vi "Data Thread.vi"() -> ()   [LabVIEW 2016]
doc: "数据处理线程；\n硬件采集的原始数据经DAQData数据队列传输至此线程，计算后获得所有物理通道数据、虚拟通道数据，再分发给显示线程数据队列（DispDATA）以及存储线程数据队列（SaveDATA）"
uses:
  ToolKit/Formula/Ctrls/PSFormula_FOR_Formula Node.ctl
  ToolKit/Formula/Ctrls/PSFormula_FOR_Formula Step.ctl
  ToolKit/Formula/Ctrls/PSFormula_FOR_Formula Para.ctl
  ToolKit/Formula/Ctrls/PSFormula_FOR_Formula MidVar Data.ctl
  HardWare/Ctrls/HardWare _ Data Queue Manage FGV Operation.ctl
  X-DAQ Viewer/Controls/ConfigFGVCtrl.ctl
  <vilib>/Analysis/baseanly.llb/Mean (DBL).vi
  Architecture/Queue Management/ARC_Queue Create_Single.vi
  Architecture/Queue Management/ARC_Queue Remove Element.vi
  Architecture/Queue Management/ARC_Queue Valid.vi
  Ctrls/GlobeVaribles.vi
  Architecture/Queue Management/ARC_Queue Insert Element.vi
  <vilib>/Utility/error.llb/DialogType.ctl
  <vilib>/Analysis/NI_AALBase.lvlib
panel:
  in  "Parameter":cluster{"Q-Local":string, "Variant":variant}
  in  "TempVariable":T5
  out "Error Report":string
  out "Current State":string
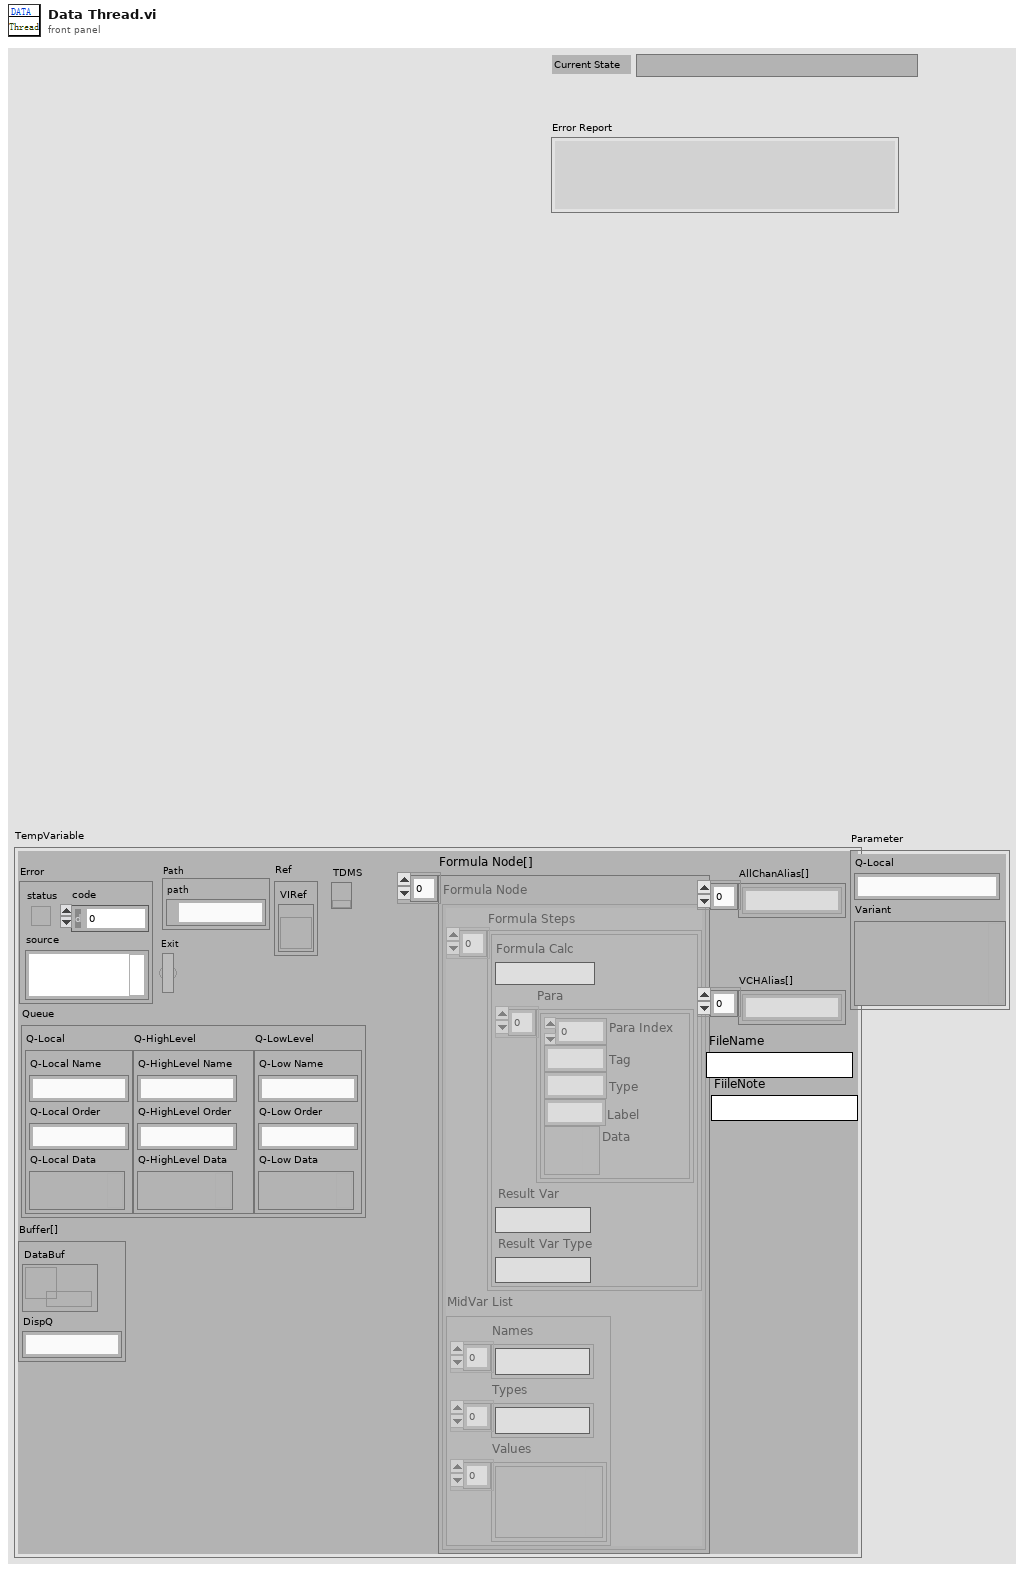
[diagram p1: front panel]
types:
  T1 = typedef "PSFormula_FOR_Formula Node.ctl" = cluster{"Formula Steps":T2[], "MidVar List":T4}
  T2 = typedef "PSFormula_FOR_Formula Step.ctl" = cluster{"Formula Calc":string, "Para":T3[], "Result Var":string, "Result Var Type":string}
  T3 = typedef "PSFormula_FOR_Formula Para.ctl" = cluster{"Para Index":i32, "Tag":string, "Type":string, "Label":string, "Data":variant}
  T4 = typedef "PSFormula_FOR_Formula MidVar Data.ctl" = cluster{"Names":string[], "Types":string[], "Values":variant[]}
  T5 = cluster{"Error":errorcluster, "Exit":bool, "Path":cluster{"path":path}, "Ref":cluster{"VIRef":refnum<vi>}, "Queue":cluster{"Q-Local":cluster{"Q-Local Name":string, "Q-Local Order":string, "Q-Local Data":variant}, "Q-HighLevel":cluster{"Q-HighLevel Name":string, "Q-HighLevel Order":string, "Q-HighLevel Data":variant}, "Q-LowLevel":cluster{"Q-Low Name":string, "Q-Low Order":string, "Q-Low Data":variant}}, "Formula Node[]":T1[], "Buffer[]":cluster{"DataBuf":refnum<queue>, "DispQ":string}, "TDMS":refnum<k34>, "AllChanAlias[]":string[], "VCHAlias[]":string[], "FileName":string, "FiileNote":string}
  T6 = cluster{"LocalName":string, "DataBuf":refnum<queue>}
  T7 = typedef "ConfigFGVCtrl.ctl" = enum16{"Initialize", "Get Value", "Set Value", "Search Info"}
  T8 = typedef "HardWare _ Data Queue Manage FGV Operation.ctl" = enum16{"Initialize", "Add", "Read", "All"}
  T9 = enum16{"Obtain Notifier", "Send Notification", "Wait Notification", "Release Notifier"}
  T10 = typedef "DialogType.ctl" = u16
  T11 = typedef "HardWare _ Channel Info.ctl" = cluster{"PhyCHtags[]":string[], "VCHTags":string[], "AllNames":string[], "AllAlias":string[], "AllUnits":string[], "AllName(Unit)":string[], "AllAlarmMax":dbl[], "AllAlarmMin":dbl[], "VCHFormula[]":string[], "VCHAlias[]":string[]}
  T12 = cluster{"PhyCHtags[]":string[], "AllAlias":string[]}
  T13 = typedef "Continuous Operations.ctl" = enum16{"Writting", "Pause", "Stop"}
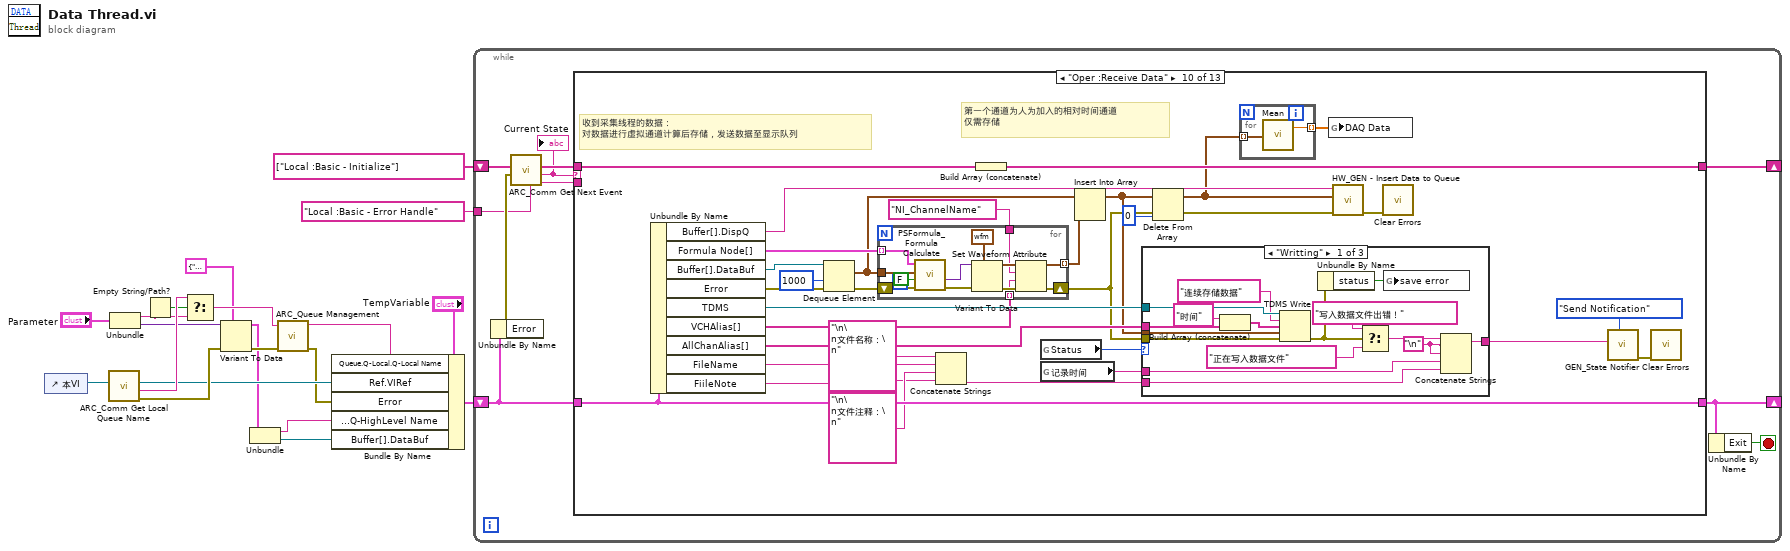
[diagram p0: block diagram]
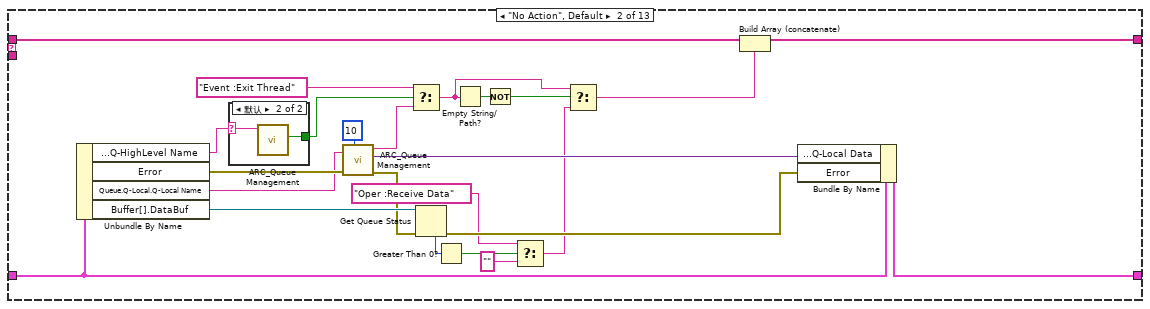
[diagram p3: hidden frame]
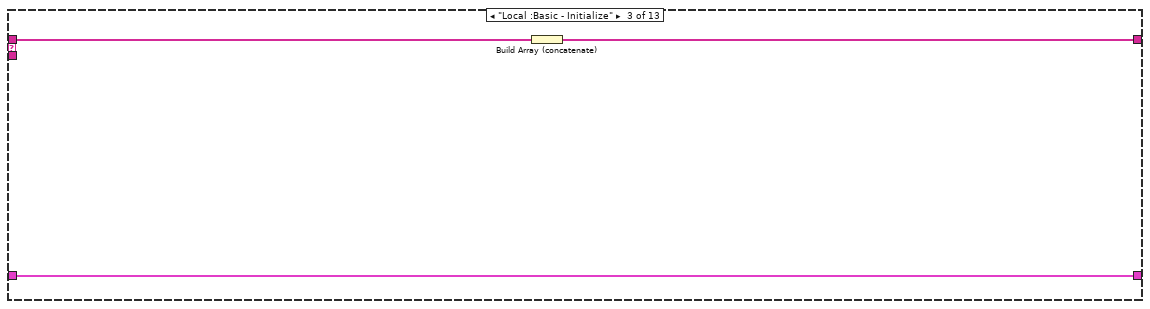
[diagram p5: hidden frame]
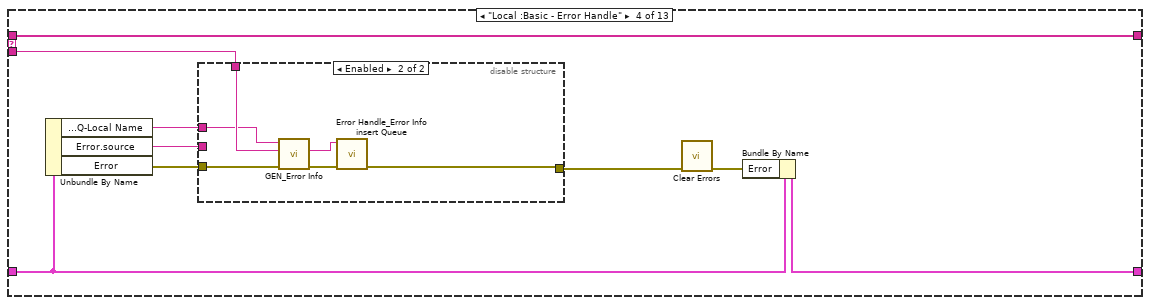
[diagram p6: hidden frame]
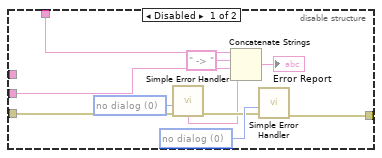
[diagram p7: hidden frame]
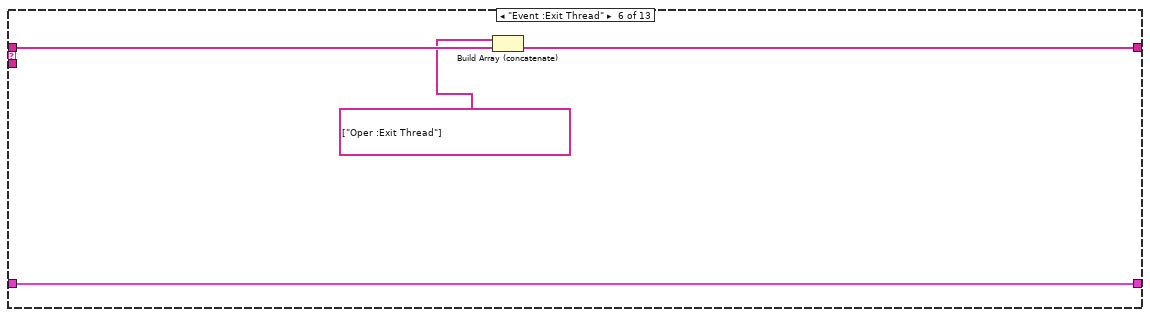
[diagram p9: hidden frame]
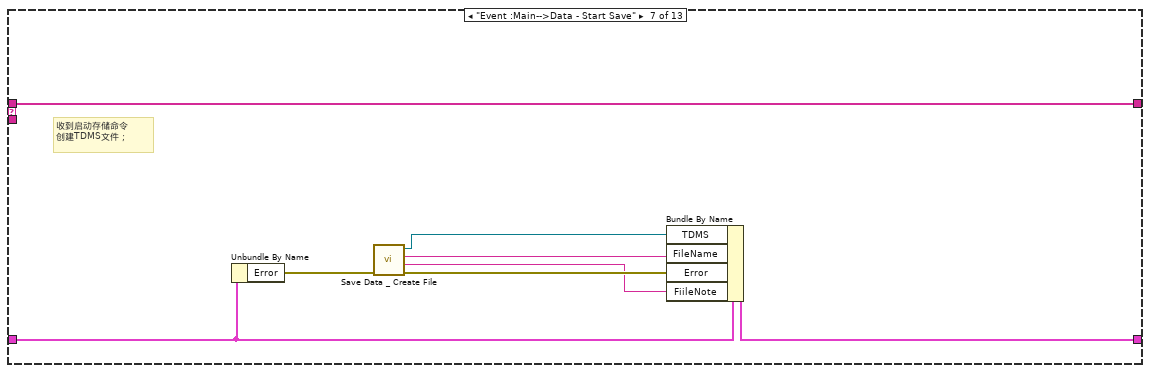
[diagram p10: hidden frame]
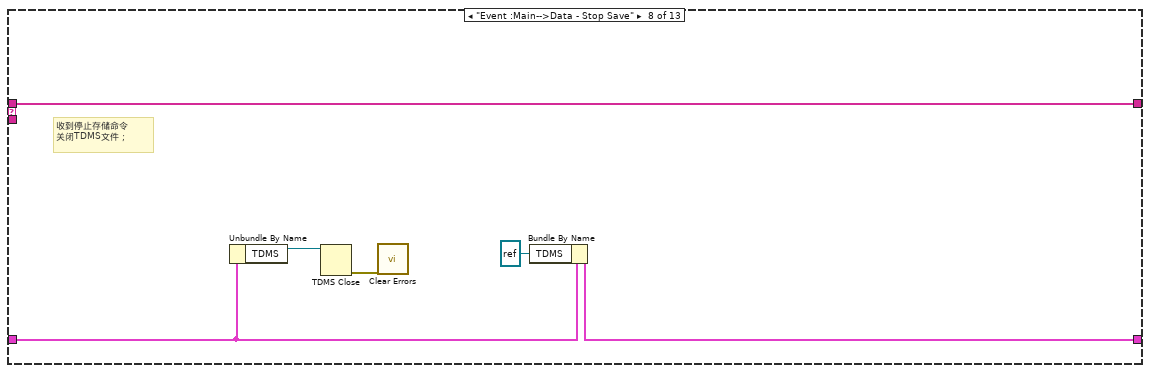
[diagram p11: hidden frame]
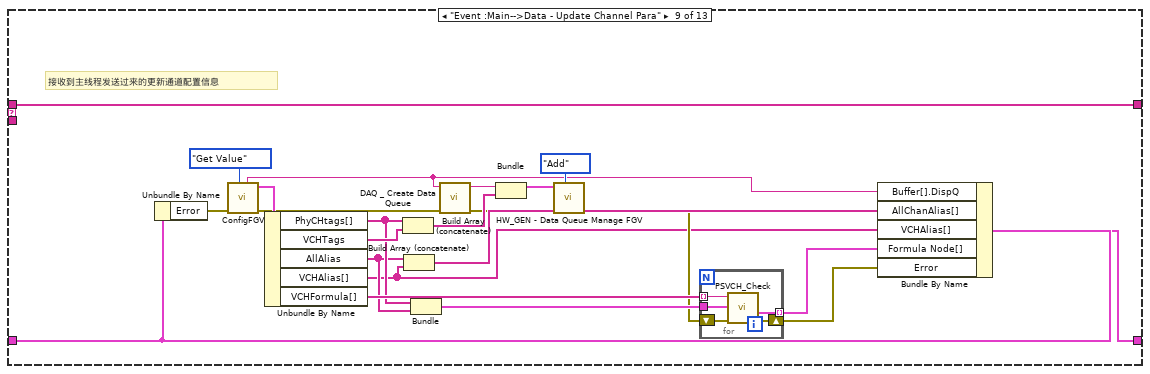
[diagram p12: hidden frame]
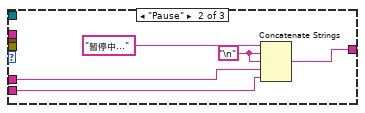
[diagram p13: hidden frame]
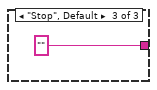
[diagram p14: hidden frame]
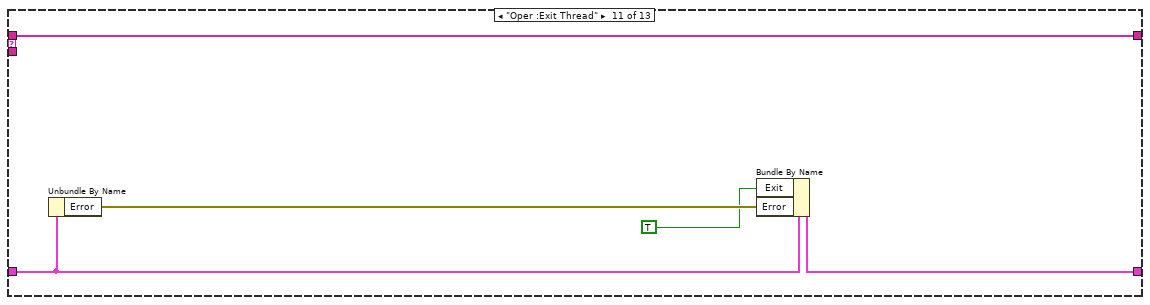
[diagram p15: hidden frame]
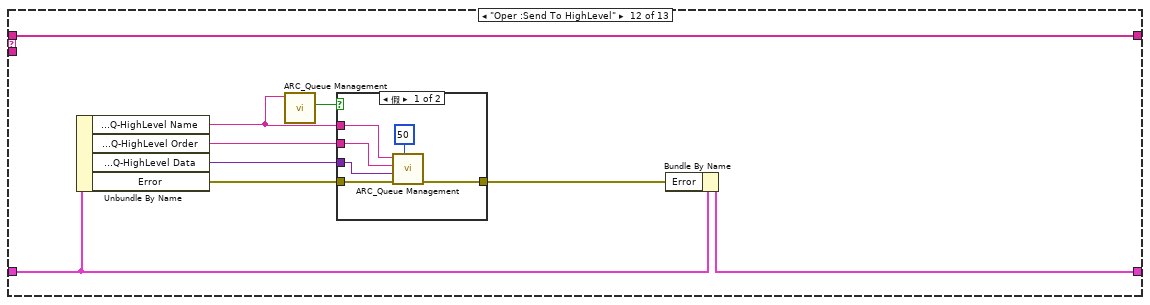
[diagram p16: hidden frame]
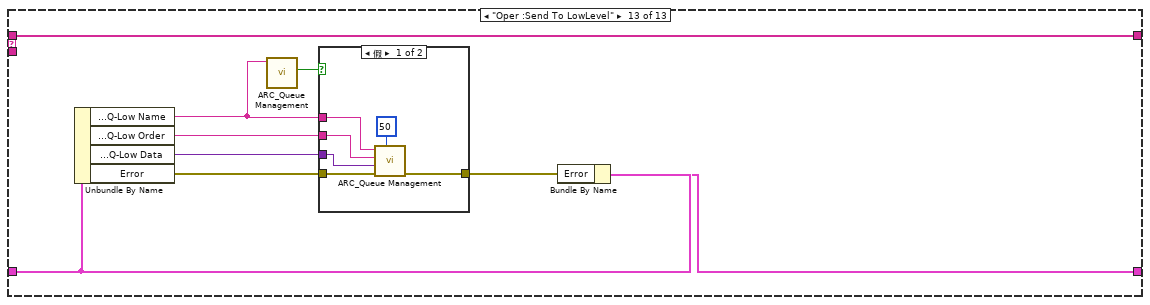
[diagram p18: hidden frame]
diagram:
  n1 = control-ref of="本VI"() -> (w12:refnum<vi>)
  n2 = call "ARC_Comm Get Local Queue Name.vi"("VI Ref"=w12) -> ("error out"=w13:errorcluster, "VI  Name"=w18:string, "VI Ref out"=w10:refnum<vi>)  [unwired: 8 in]
  n3 = Unbundle("Parameter") -> ("Q-Local"=w14:string, "Variant"=w17:variant)
  n4 = Empty String/Path?(string/path=w14) -> (empty?=w16:bool)
  n5 = Select(t=w18, s=w16, f=w14) -> (s? t:f=w7:string)
  n6 = Variant To Data(error in=w13, type=T6 {"LocalName"="", "DataBuf"=refnum} ("output cluster"), Variant=w17) -> (data=w3:T6, error out=w11:errorcluster)
  n7 = Unbundle(w3) -> ("LocalName"=w2:string, "DataBuf"=w1:refnum<queue>)
  n8 = call-poly "ARC_Queue Management.vi"("error in"=w11, "Queue Name"=w7) -> ("error out"=w9:errorcluster, "Queue Name dup"=w8:string)  [unwired: 7 in, 1 out]
  n9 = Bundle By Name(cluster="TempVariable", "Queue.Q-Local.Q-Local Name"=w8, "Ref.VIRef"=w10, "Error"=w9, "Queue.Q-HighLevel.Q-HighLevel Name"=w2, "Buffer[].DataBuf"=w1) -> (w5:T5)
  n10 = while {
    shift-right: [w25] -> _
    shift-left: w5 -> [w27]
    shift-right: [w28] -> _
    shift-left: string[] ["Local :Basic - Initialize"] ("event queue out") -> [w30]
    tunnel: "Local :Basic - Error Handle" ("Error Handle") -> [w24]
    stop <- w21 stop-if-true
    n11 = Unbundle By Name(w27) -> ("Error"=w26:errorcluster)
    n12 = call "ARC_Comm Get Next Event.vi"("Error Handle"=w24, "error in (no error)"=w26, "event queue in"=w30) -> ("prev event"=w23:string, "next event"=w22:string, "event queue out"=w29:string[])  [unwired: 3 in]
    "Current State" <- w22
    n13 = case shown="\"Oper :Receive Data\"" w22 {
      tunnel: w27 -> [w31 w56 w59 w68 w87 w91 w99 w105 w128 w163 w204 w213 w229]
      tunnel: w29 -> [w32 w50 w61 w70 w88 w92 w100 w106 w129 w165 w207 w216 w232]
      tunnel: [w32 w49 w60 w70 w88 w90 w100 w106 w129 w164 w207 w216 w232] -> w28
      tunnel: [w31 w55 w59 w69 w87 w91 w97 w104 w124 w163 w205 w212 w228] -> w25
      tunnel: w23 -> [_ _ _ w65 _ _ _ _ _ _ _ _ _]
      frame "----------Core Status----------" {
      }
      frame "No Action", Default {
        n14 = Unbundle By Name(w56) -> ("Queue.Q-HighLevel.Q-HighLevel Name"=w52:string, "Error"=w53:errorcluster, "Queue.Q-Local.Q-Local Name"=w51:string, "Buffer[].DataBuf"=w44:refnum<queue>)
        n15 = case shown="默认" w52 {
          selector: w52 -> [_ w57]
          tunnel: [_ w58] -> w45
          frame "" {
          }
          frame Default {
            n16 = call-poly "ARC_Queue Management.vi"("Queue Name(unamed)"=w57) -> ("Not Exist?"=w58:bool)  [unwired: 8 in, 2 out]
          }
        }
        n17 = call-poly "ARC_Queue Management.vi"("Time out(-1)_queue out"=10, "error in (no error)"=w53, "Queue Name(unamed)"=w51) -> ("error out"=w41:errorcluster, "Data"=w54:variant, "Event"=w46:string)  [unwired: 5 in, 1 out]
        n18 = Select(t="Event :Exit Thread" ("Event"), s=w45, f=w46) -> (s? t:f=w37:string)
        n19 = Get Queue Status(queue=w44, error in (no error)=w41) -> (error out=w40:errorcluster, # elements in queue=w43:i32)  [unwired: 1 in, 6 out]
        n20 = Greater Than 0?(x=w43) -> (x > 0?=w42:bool)
        n21 = Empty String/Path?(string/path=w37) -> (empty?=w39:bool)
        n22 = Not(x=w39) -> (.not. x?=w38:bool)
        n23 = Select(t="Oper :Receive Data" ("Event"), s=w42, f="") -> (s? t:f=w36:string)
        n24 = Select(t=w37, s=w38, f=w36) -> (s? t:f=w35:string)
        n25 = Build Array (concatenate)(w50, w35) -> (w49:string[])
        n26 = Bundle By Name(cluster=w56, "Queue.Q-Local.Q-Local Data"=w54, "Error"=w40) -> (w55:T5)
      }
      frame "Local :Basic - Initialize" {
        n27 = Build Array (concatenate)(w61) -> (w60:string[])
      }
      frame "Local :Basic - Error Handle" {
        n28 = Unbundle By Name(w68) -> ("Queue.Q-Local.Q-Local Name"=w62:string, "Error.source"=w64:string, "Error"=w66:errorcluster)
        n29 = disable-structure shown="Enabled" {
          disable-tunnel: w66 -> [w80 w84]
          disable-tunnel: w65 -> [w79 w82]
          disable-tunnel: w64 -> [w78 _]
          disable-tunnel: [w77 w83] -> w63
          disable-tunnel: w62 -> [_ w81]
          frame Disabled {
            w74 = T10 0 items=["no dialog", "OK message", "continue or stop message", "OK message + warnings", "continue/stop + warnings"] ("type of dialog (OK msg:1)")
            w76 = T10 0 items=["no dialog", "OK message", "continue or stop message", "OK message + warnings", "continue/stop + warnings"] ("type of dialog (OK msg:1)")
            n30 = call <vilib>:"Simple Error Handler.vi"("type of dialog (OK msg:1)"=w74, "error in (no error)"=w80) -> ("error out"=w75:errorcluster, "message"=w72:string)  [unwired: 3 in, 3 out]
            n31 = Concatenate Strings(w79, " -> " ("字符串"), w78, w72) -> (→"Error Report":string)
            n32 = call <vilib>:"Simple Error Handler.vi"("type of dialog (OK msg:1)"=w76, "error in (no error)"=w75) -> ("error out"=w77:errorcluster)  [unwired: 3 in, 4 out]
          }
          frame Enabled {
            n33 = call "GEN_Error Info.vi"("error in"=w84, "Event name"=w82, "Thread name"=w81) -> ("error out"=w85:errorcluster, "Error Report"=w86:string)  [unwired: 7 in]
            n34 = call "Error Handle_Error Info insert Queue.vi"("error in"=w85, "error info in"=w86) -> ("error out"=w83:errorcluster)  [unwired: 9 in]
          }
        }
        n35 = call <vilib>:"Clear Errors.vi"("error in (no error)"=w63) -> ("error out"=w67:errorcluster)  [unwired: 5 in, 1 out]
        n36 = Bundle By Name(cluster=w68, "Error"=w67) -> (w69:T5)
      }
      frame "----------event----------" {
      }
      frame "Event :Exit Thread" {
        n37 = Build Array (concatenate)(string[] ["Oper :Exit Thread"] ("数组"), w92) -> (w90:string[])
      }
      frame "Event :Main-->Data - Start Save" {
        # "收到启动存储命令\n创建TDMS文件；"
        n38 = Unbundle By Name(w99) -> ("Error"=w98:errorcluster)
        n39 = call "Save Data _ Create File.vi"("error in"=w98) -> ("error out"=w96:errorcluster, "FiileNote"=w93:string, "FileName"=w94:string, "file out"=w95:refnum<k34>)  [unwired: 7 in]
        n40 = Bundle By Name(cluster=w99, "TDMS"=w95, "FileName"=w94, "Error"=w96, "FiileNote"=w93) -> (w97:T5)
      }
      frame "Event :Main-->Data - Stop Save" {
        # "收到停止存储命令\n关闭TDMS文件；"
        n41 = Unbundle By Name(w105) -> ("TDMS"=w103:refnum<k34>)
        n42 = TDMS Close(11:w103) -> (0:w102:errorcluster)  [unwired: 1 in, 1 out]
        n43 = call <vilib>:"Clear Errors.vi"("error in (no error)"=w102) -> ()  [unwired: 5 in, 2 out]
        n44 = Bundle By Name(cluster=w105, "TDMS"=refnum<k34> refnum) -> (w104:T5)
      }
      frame "Event :Main-->Data - Update Channel Para" {
        # "接收到主线程发送过来的更新通道配置信息"
        n45 = Unbundle By Name(w128) -> ("Error"=w117:errorcluster)
        n46 = call "ConfigFGV.vi"("Command"=ConfigFGVCtrl."Get Value", "error in"=w117) -> ("error out"=w116:errorcluster, "CHInfoOut"=w121:T11, "DevName"=w122:string)  [unwired: 5 in, 2 out]
        n47 = Unbundle By Name(w121) -> ("PhyCHtags[]"=w112:string[], "VCHTags"=w120:string[], "AllAlias"=w111:string[], "VCHAlias[]"=w108:string[], "VCHFormula[]"=w115:string[])
        n48 = Build Array (concatenate)(w112, w120) -> (w119:string[])
        n49 = Build Array (concatenate)(w111, w108) -> (w118:string[])
        n50 = Bundle("PhyCHtags[]"=w112, "AllAlias"=w111) -> (w110:T12)  [unwired: 1 in]
        n51 = call "DAQ _ Create Data Queue.vi"("error in"=w116, "Q-name"=w122) -> ("error out"=w114:errorcluster, "queue name"=w126:string)  [unwired: 8 in]
        n52 = Bundle("queue name"=w126, w119) -> (w125:cluster{"queue name":string, string[]})  [unwired: 1 in]
        n53 = call "HW_GEN - Data Queue Manage FGV.vi"("Oper."=HardWare___Data_Queue_Manage_FGV_Operation."Add", "error in"=w114, "Add Chan"=w125) -> ("error out"=w109:errorcluster)  [unwired: 6 in, 2 out]
        n54 = for {
          tunnel: w115 -> [w134] mode=indexing
          shift-right: [w132] -> w107
          shift-left: w109 -> [w133]
          tunnel: [w131] -> w113 mode=indexing
          tunnel: w110 -> [w130]
          n55 = call "PSVCH_Check.vi"("Error In (no error)"=w133, "VarList"=w130, "Formula"=w134) -> ("Error Out"=w132:errorcluster, "Formula Node out"=w131:T1)  [unwired: 4 in, 3 out]
        }
        n56 = Bundle By Name(cluster=w128, "Buffer[].DispQ"=w122, "AllChanAlias[]"=w118, "VCHAlias[]"=w108, "Formula Node[]"=w113, "Error"=w107) -> (w124:T5)
      }
      frame "Oper :Receive Data" {
        # "第一个通道为人为加入的相对时间通道\n仅需存储"
        # "收到采集线程的数据：\n对数据进行虚拟通道计算后存储，发送数据至显示队列"
        n57 = Unbundle By Name(w163) -> ("Buffer[].DispQ"=w155:string, "Formula Node[]"=w158:T1[], "Buffer[].DataBuf"=w161:refnum<queue>, "Error"=w162:errorcluster, "TDMS"=w154:refnum<k34>, "VCHAlias[]"=w148:string[], "AllChanAlias[]"=w153:string[], "FileName"=w144:string, "FiileNote"=w138:string)
        n58 = Dequeue Element(queue=w161, timeout in ms (-1)=1000, error in (no error)=w162) -> (element=w156:waveform(dbl)[], error out=w159:errorcluster)  [unwired: 2 out]
        n59 = for {
          shift-right: [w192] -> w152
          shift-left: w159 -> [w200]
          tunnel: w158 -> [w202] mode=indexing
          tunnel: w156 -> [w199]
          tunnel: [w194] -> w157 mode=indexing
          tunnel: "NI_ChannelName" ("name") -> [w191]
          tunnel: w148 -> [w190] mode=indexing
          n60 = call "PSFormula_Formula Calculate.vi"("error in"=w200, "Complex Variable(T)"=FALSE, "Values"=w199, "Formula Node"=w202) -> ("error out"=w196:errorcluster, "Value"=w197:variant)  [unwired: 4 in, 2 out]
          n61 = Variant To Data(error in=w196, type=waveform(dbl) {"t0"=timestamp(0 s since 1904-01-01), "dt"=1.0, "Y"=[]} ("Waveform"), Variant=w197) -> (data=w195:waveform(dbl), error out=w193:errorcluster)
          n62 = Set Waveform Attribute(4:w193, 5:w190, 6:w191, 7:w195) -> (0:w192:errorcluster, 3:w194:waveform(dbl))  [unwired: 1 out]
        }
        n63 = Concatenate Strings("\n\n文件名称：\n" ("字符串"), w144, "\n\n文件注释：\n" ("字符串"), w138) -> (w143:string)
        n64 = Build Array (concatenate)(w165) -> (w164:string[])
        n65 = global read "GlobeVaribles.vi" "Status"() -> (w151:T13)
        n66 = global read "GlobeVaribles.vi" "记录时间"() -> (w135:string)
        n67 = Insert Into Array(array=w156, new element=w157) -> (w141:waveform(dbl)[])  [unwired: 1 in]
        n68 = case shown="\"Writting\"" w151 {
          tunnel: w154 -> [w183 _ _]
          tunnel: w141 -> [w182 _ _]
          tunnel: w153 -> [w172 _ _]
          tunnel: w152 -> [w174 _ _]
          tunnel: [w178 w187 "" ("组名称输入（无标题）")] -> w146
          tunnel: w143 -> [w177 w186 _]
          tunnel: w135 -> [w169 w185 _]
          frame "Writting" {
            w168 = "\n"
            n69 = Build Array (concatenate)("时间" ("组名称输入（无标题）"), w172) -> (w171:string[])
            n70 = TDMS Write(0:w183, 5:"连续存储数据" ("组名称输入（无标题）"), 7:w171, 9:w182, 11:w174) -> (15:w176:errorcluster)  [unwired: 1 in, 3 out]
            n71 = Unbundle By Name(w176) -> ("status"=w175:bool)
            n72 = Select(t="写入数据文件出错！" ("组名称输入（无标题）"), s=w176, f="正在写入数据文件" ("组名称输入（无标题）")) -> (s? t:f=w179:string)
            n73 = global write "GlobeVaribles.vi" "save error"(w175) -> ()
            n74 = Concatenate Strings(w179, w168, w168, w169, w177) -> (w178:string)
          }
          frame "Pause" {
            w184 = "\n"
            n75 = Concatenate Strings("暂停中..." ("组名称输入（无标题）"), w184, w184, w185, w186) -> (w187:string)
          }
          frame "Stop", Default {
          }
        }
        n76 = Delete From Array(array=w141, index=0 ("长度")) -> (array with subset deleted=w136:waveform(dbl)[])  [unwired: 1 in, 1 out]
        n77 = for {
          tunnel: w136 -> [w167] mode=indexing
          tunnel: [w166] -> w140 mode=indexing
          n78 = call-poly <vilib>:"Mean.vi"("X"=w167) -> ("mean"=w166:dbl)  [unwired: 1 out]
        }
        n79 = global write "GlobeVaribles.vi" "DAQ Data"(w140) -> ()
        n80 = call "HW_GEN - Insert Data to Queue.vi"("error in"=w152, "data"=w136, "Object Name"=w155) -> ("error out"=w150:errorcluster)  [unwired: 7 in, 1 out]
        n81 = call <vilib>:"Clear Errors.vi"("error in (no error)"=w150) -> ()  [unwired: 5 in, 2 out]
        n82 = call "GEN_State Notifier.vi"("Action Select"=T9."Send Notification", "Notification"=w146) -> ("error out"=w145:errorcluster)  [unwired: 8 in, 1 out]
        n83 = call <vilib>:"Clear Errors.vi"("error in (no error)"=w145) -> ()  [unwired: 5 in, 2 out]
      }
      frame "Oper :Exit Thread" {
        n84 = Unbundle By Name(w204) -> ("Error"=w206:errorcluster)
        n85 = Bundle By Name(cluster=w204, "Exit"=TRUE, "Error"=w206) -> (w205:T5)
      }
      frame "Oper :Send To HighLevel" {
        n86 = Unbundle By Name(w213) -> ("Queue.Q-HighLevel.Q-HighLevel Name"=w215:string, "Queue.Q-HighLevel.Q-HighLevel Order"=w210:string, "Queue.Q-HighLevel.Q-HighLevel Data"=w209:variant, "Error"=w214:errorcluster)
        n87 = call-poly "ARC_Queue Management.vi"("Queue Name(unamed)"=w215) -> ("Not Exist?"=w211:bool)  [unwired: 8 in, 2 out]
        n88 = case shown="假" w211 {
          tunnel: w214 -> [w222 w223]
          tunnel: w215 -> [w220 _]
          tunnel: w210 -> [w218 _]
          tunnel: w209 -> [w219 _]
          tunnel: [w217 w223] -> w208
          frame False {
            n89 = call-poly "ARC_Queue Management.vi"("Time out(-1)_queue in"=50, "error in (no error)"=w222, "Data"=w219, "Event"=w218, "Queue Name(unamed)"=w220) -> ("error out"=w217:errorcluster)  [unwired: 5 in, 1 out]
          }
          frame True {
          }
        }
        n90 = Bundle By Name(cluster=w213, "Error"=w208) -> (w212:T5)
      }
      frame "Oper :Send To LowLevel" {
        n91 = Unbundle By Name(w229) -> ("Queue.Q-LowLevel.Q-Low Name"=w231:string, "Queue.Q-LowLevel.Q-Low Order"=w226:string, "Queue.Q-LowLevel.Q-Low Data"=w225:variant, "Error"=w230:errorcluster)
        n92 = call-poly "ARC_Queue Management.vi"("Queue Name(unamed)"=w231) -> ("Not Exist?"=w227:bool)  [unwired: 8 in, 2 out]
        n93 = case shown="假" w227 {
          tunnel: w230 -> [w238 w239]
          tunnel: w231 -> [w236 _]
          tunnel: w226 -> [w234 _]
          tunnel: w225 -> [w235 _]
          tunnel: [w233 w239] -> w224
          frame False {
            n94 = call-poly "ARC_Queue Management.vi"("Time out(-1)_queue in"=50, "error in (no error)"=w238, "Data"=w235, "Event"=w234, "Queue Name(unamed)"=w236) -> ("error out"=w233:errorcluster)  [unwired: 5 in, 1 out]
          }
          frame True {
          }
        }
        n95 = Bundle By Name(cluster=w229, "Error"=w224) -> (w228:T5)
      }
    }
    n96 = Unbundle By Name(w25) -> ("Exit"=w21:bool)
  }
